vi "Default Counter Channels.vi"(1 "Channels":T7={"# Input Channels"=0, "# Output Channels"=0, "Channel Type"=enum."Digital", "Units"=""}) -> (0 "Counter":T1 {"Counter Channels"."Frequency Measurement"."Measurement Timebase" items=["256 us", "512 us", "1024 us", "2048 us", "4096 us", "8192 us", "16384 us", "32768 us"]; "Counter Channels"."Frequency Measurement"."Measurement Edge" items=["Rising Edge", "Falling Edge"]; "Counter Channels"."Pulse Width Measurement"."Measurement Type" items=["High Pulse"=3, "Low Pulse"=4, "Most Recent"=5]; "Counter Channels"."Period Measurement"."Measurement Edge" items=["Rising Edge", "Falling Edge"]; "Counter Channels"."Count Edges"."Gate Mode" items=["Next Channel"=1, "Always Enabled"=3]; "Counter Channels"."Count Edges"."Output Mode" items=["Toggle, Reset Off", "Toggle, Reset On", "On Pulse", "Off Pulse"]; "Counter Channels"."Count Edges"."Counter Direction" items=["Count up", "Count down"]; "Counter Channels"."Count Edges"."Counter Source" items=["This Channel", "Terminal count of previous channel"]; "Counter Channels"."Count Edges"."Counter Event" items=["Rising Edge", "Falling Edge", "Any Edge"]; "Counter Channels"."Measurement Mode" items=["Count Edges", "Period Measurements", "Pulse Width Measurements", "Frequency Measurements"]})   [LabVIEW 2020, in "Modules.lvlib" / "SD Module.lvclass"]
uses:
  SD Module.lvclass
  RSI Module/Channels.ctl
  RSI Module/Channel Type.ctl
  Type Defs/Counter.ctl
  Type Defs/Counter Channel.ctl
  Type Defs/Count Edges.ctl
  Type Defs/Period Measurement.ctl
  Type Defs/Pulse Width Measurement.ctl
  Type Defs/Frequency Measurement.ctl
  RSI Module/RSI Module.lvclass
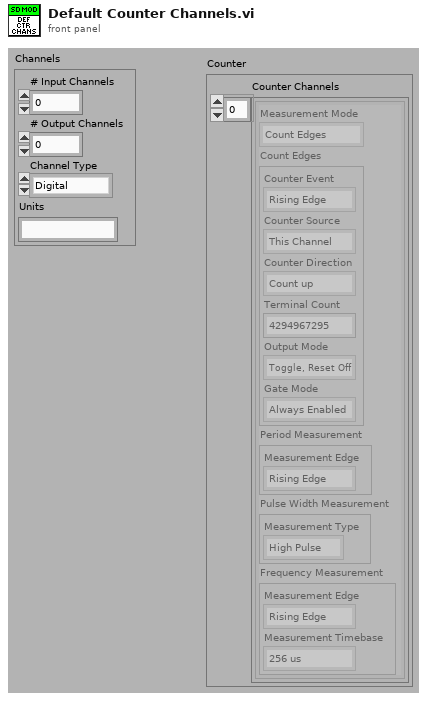
[diagram p1: front panel]
types:
  T1 = typedef "Modules.lvlib/SD Module.lvclass/Counter.ctl" = cluster{"Counter Channels":T2[]}
  T2 = typedef "Modules.lvlib/SD Module.lvclass/Counter Channel.ctl" = cluster{"Measurement Mode":u32, "Count Edges":T3, "Period Measurement":T4, "Pulse Width Measurement":T5, "Frequency Measurement":T6}
  T3 = typedef "Modules.lvlib/SD Module.lvclass/Count Edges.ctl" = cluster{"Counter Event":u32, "Counter Source":u32, "Counter Direction":u32, "Terminal Count":u32, "Output Mode":u32, "Gate Mode":u32}
  T4 = typedef "Modules.lvlib/SD Module.lvclass/Period Measurement.ctl" = cluster{"Measurement Edge":u32}
  T5 = typedef "Modules.lvlib/SD Module.lvclass/Pulse Width Measurement.ctl" = cluster{"Measurement Type":u32}
  T6 = typedef "Modules.lvlib/SD Module.lvclass/Frequency Measurement.ctl" = cluster{"Measurement Edge":u32, "Measurement Timebase":u32}
  T7 = typedef "Modules.lvlib/RSI Module.lvclass/Channels.ctl" = cluster{"# Input Channels":i32, "# Output Channels":i32, "Channel Type":T8, "Units":string}
  T8 = typedef "Modules.lvlib/RSI Module.lvclass/Channel Type.ctl" = enum16{"Analog", "Digital"}
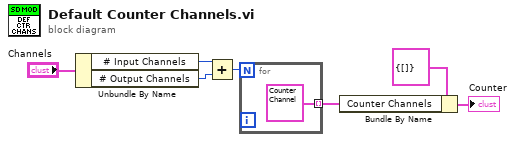
[diagram p0: block diagram]
diagram:
  n1 = Unbundle By Name("Channels") -> ("# Input Channels"=w3:i32, "# Output Channels"=w2:i32)
  n2 = Add(x=w3, y=w2) -> (x+y=w1:i32)
  n3 = for {
    N: w1 -> [_]
    tunnel: [T2 {"Measurement Mode"=0, "Count Edges"={"Counter Event"=0, "Counter Source"=0, "Counter Direction"=0, "Terminal Count"=4294967295, "Output Mode"=0, "Gate Mode"=3}, "Period Measurement"={"Measurement Edge"=0}, "Pulse Width Measurement"={"Measurement Type"=3}, "Frequency Measurement"={"Measurement Edge"=0, "Measurement Timebase"=0}} ("Counter Channel")] -> w5 mode=indexing
  }
  n4 = Bundle By Name(cluster=T1 {"Counter Channels"=[]} ("Counter"), "Counter Channels"=w5) -> (→"Counter":T1)
